vi "Set Number of Slots.vi"(8 "error in":errorcluster, 10 "number of slots":i32, 11 "chassis ref in":T1 format="%.0x") -> (0 "error out":errorcluster, 3 "chassis ref out":T1 format="%.0x")   [LabVIEW 2020, in "Scan Engine Scripting.lvlib"]
doc: "Writes <B>number of slots</B> into the provided chassis reference and edits the existing slots of the chassis to comply with the new limit."
uses:
  Scan Engine Scripting.lvlib
  <vilib>/NI VeriStand/Custom Device API/Custom Device Item Ref.ctl
  Modules.lvlibp/RSI Module/Slot Settings.ctl
  Modules.lvlibp/RSI Module/Module Models.ctl
  Scan Engine Dependencies.llb/Scan Engine GUIDs.vi
  Modules.lvlibp/RSI Module/Class Property Strings.vi
  Scan Engine Dependencies.llb/Property Strings.vi
  <vilib>/NI VeriStand/Custom Device API/Set Item Property (I32).vi
  Scan Engine Dependencies.llb/Scan Engine Custom Device.lvlib
  <vilib>/NI VeriStand/Custom Device API/Custom Device API.lvlib
  Modules.lvlibp/RSI Module/RSI Module.lvclass
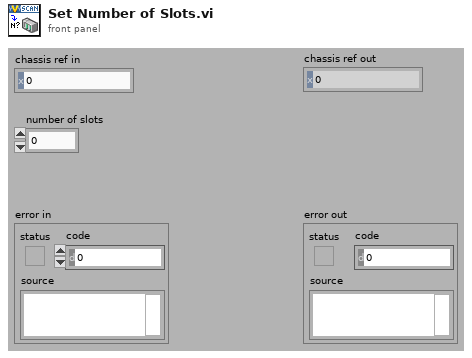
[diagram p1: front panel]
types:
  T1 = typedef "Custom Device API.lvlib/Custom Device Item Ref.ctl" = u64
  T2 = typedef "Modules.lvlibp/RSI Module.lvclass/Module Models.ctl" = enum16{"Empty", "NI 9201", "NI 9203", "NI 9205", "NI 9206", "NI 9207", "NI 9208", "NI 9209", "NI 9210", "NI 9211", "NI 9212", "NI 9213", "NI 9214", "NI 9215", "NI 9216", "NI 9217", "NI 9219", "NI 9220", "NI 9221", "NI 9222", "NI 9223", "NI 9224", "NI 9225", "NI 9226", "NI 9227", "NI 9228", "NI 9229", "NI 9233", "NI 9234", "NI 9235", "NI 9236", "NI 9237", "NI 9239", "NI 9242", "NI 9244", "NI 9253", "NI 9263", "NI 9264", "NI 9265", "NI 9266", "NI 9269", "NI 9344", "NI 9350", "NI 9375", "NI 9401", "NI 9402", "NI 9403", "NI 9411", "NI 9421", "NI 9422", "NI 9423", "NI 9425", "NI 9426", "NI 9435", "NI 9436", "NI 9437", "NI 9472", "NI 9474", "NI 9475", "NI 9476", "NI 9477", "NI 9478", "NI 9481", "NI 9482", "NI 9485"}
  T3 = typedef "Modules.lvlibp/RSI Module.lvclass/Slot Settings.ctl" = cluster{"Slot":u32, "EtherCAT?":bool}
  T4 = typedef "Custom Device API.lvlib/Custom Device Item Info.ctl" = cluster{"Name":string, "Is Channel":bool, "GUID":string, "Is Waveform":bool}
  T5 = typedef "Modules.lvlibp/Custom Device API.lvlib/Custom Device Item Ref.ctl" = u64
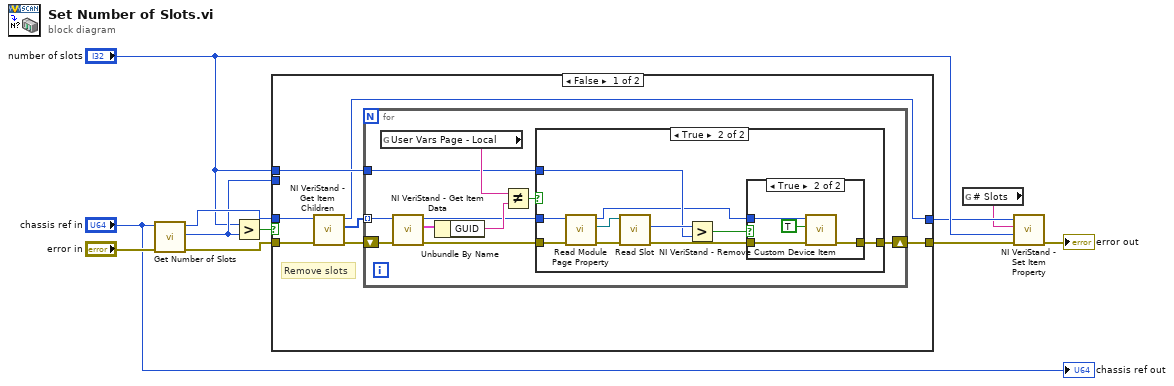
[diagram p0: block diagram]
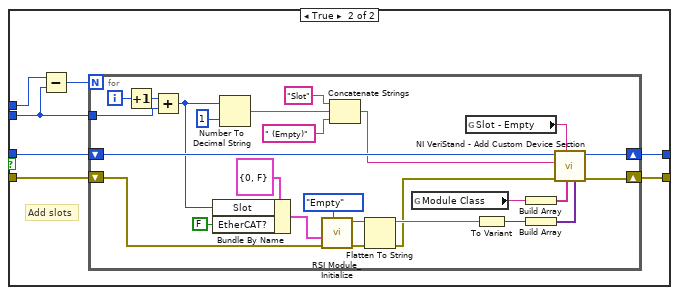
[diagram p4: hidden frame]
diagram:
  n1 = call "Get Number of Slots.vi"("error in"="error in", "chassis ref in"="chassis ref in") -> ("error out"=w11:errorcluster, "number of slots"=w7:i32, "chassis ref out"=w10:T1)  [unwired: 7 in]
  n2 = Greater?(x="number of slots", y=w7) -> (0:w9:bool)
  n3 = case shown="False" w9 {
    tunnel: w10 -> [w18 w47]
    tunnel: w11 -> [w17 w50]
    tunnel: [w14 w46] -> w6
    tunnel: "number of slots" -> [w13 w51]
    tunnel: w7 -> [_ w48]
    tunnel: [w12 w45] -> w3
    frame False {
      # "Remove slots"
      n4 = call <vilib>:"NI VeriStand - Get Item Children.vi"("error in (no error)"=w17, "Item Ref in"=w18) -> ("error out"=w15:errorcluster, "Child Refs"=w16:T1[], "Item Ref out"=w12:T1)  [unwired: 6 in, 1 out]
      n5 = for {
        tunnel: w16 -> [w27] mode=indexing
        shift-right: [w19] -> w14
        shift-left: w15 -> [w28]
        tunnel: w13 -> [w20]
        n6 = global read "Scan Engine GUIDs.vi" "User Vars Page - Local"() -> (w24:string)
        n7 = call <vilib>:"NI VeriStand - Get Item Data.vi"("error in (no error)"=w28, "Item Ref in"=w27) -> ("error out"=w21:errorcluster, "Item Info"=w26:T4, "Item Ref out"=w22:T1)  [unwired: 6 in, 1 out]
        n8 = Unbundle By Name(w26) -> ("GUID"=w25:string)
        n9 = Not Equal?(x=w24, y=w25) -> (x != y?=w23:bool)
        n10 = case shown="True" w23 {
          tunnel: w22 -> [_ w38]
          tunnel: w21 -> [w29 w39]
          tunnel: w20 -> [_ w34]
          tunnel: [w29 w30] -> w19
          frame False {
          }
          frame True {
            n11 = call "Read Module Page Property.vi"("error in (no error)"=w39, "Node Ptr In"=w38) -> ("error out"=w37:errorcluster, "RSI Module"=w36:refnum<class "RSI Module.lvclass">, "Node Ptr Out"=w31:T5)  [unwired: 7 in]
            n12 = call "Read Slot.vi"("error in (no error)"=w37, "RSI Module in"=w36) -> ("error out"=w32:errorcluster, "Slot"=w35:u32)  [unwired: 7 in, 1 out]
            n13 = Greater?(x=w35, y=w34) -> (0:w33:bool)
            n14 = case shown="True" w33 {
              tunnel: w32 -> [w40 w44]
              tunnel: w31 -> [_ w43]
              tunnel: [w40 w41] -> w30
              frame False {
              }
              frame True {
                n15 = call <vilib>:"NI VeriStand - Remove Custom Device Item.vi"("error in (no error)"=w44, "Force Delete (F)"=TRUE, "Item Ref in"=w43) -> ("error out"=w41:errorcluster)  [unwired: 7 in, 1 out]
              }
            }
          }
        }
      }
    }
    frame True {
      # "Add slots"
      n16 = Subtract(x=w51, y=w48) -> (x-y=w49:i32)
      n17 = for {
        N: w49 -> [_]
        shift-right: [w72] -> w46
        shift-left: w50 -> [w65]
        shift-right: [w71] -> w45
        shift-left: w47 -> [w77]
        tunnel: w48 -> [w53]
        i -> [w74]
        n18 = Increment(x=w74) -> (x+1=w54:i32)
        n19 = Add(x=w54, y=w53) -> (x+y=w52:i32)
        n20 = Bundle By Name(cluster=T3 {"Slot"=0, "EtherCAT?"=FALSE} ("Slot Settings"), "Slot"=w52, "EtherCAT?"=FALSE) -> (w68:T3)
        n21 = Number To Decimal String(number=w52, width (-)=i16 1) -> (decimal integer string=w76:string)
        n22 = call "RSI Module_Initialize.vi"("Module Model"=Module_Models."Empty" ("Module"), "error in (no error)"=w65, "Slot Settings"=w68) -> ("error out"=w58:errorcluster, "RSI Module out"=w60:refnum<class "RSI Module.lvclass">)  [unwired: 7 in]
        n23 = Concatenate Strings("Slot" ("string"), w76, " (Empty)" ("Section Name")) -> (w73:string)
        n24 = Flatten To String(anything=w60, error in (no error)=w58) -> (data string=w59:string, error out=w57:errorcluster)  [unwired: 2 in, 1 out]
        n25 = global read "Class Property Strings.vi" "Module Class"() -> (w56:string)
        n26 = global read "Scan Engine GUIDs.vi" "Slot - Empty"() -> (w61:string)
        n27 = To Variant(anything=w59) -> (Variant=w69:variant)
        n28 = Build Array(w56) -> (w64:string[])
        n29 = Build Array(w69) -> (w70:variant[])
        n30 = call <vilib>:"NI VeriStand - Add Custom Device Section.vi"("Property Values"=w70, "Property names"=w64, "GUID (Default Section)"=w61, "error in (no error)"=w57, "Section Name"=w73, "Parent Ref in"=w77) -> ("error out"=w72:errorcluster, "Parent Ref out"=w71:T1)  [unwired: 2 in, 2 out]
      }
    }
  }
  n31 = global read "Property Strings.vi" "# Slots"() -> (w2:string)
  n32 = call-poly <vilib>:"NI VeriStand - Set Item Property.vi"("error in (no error)"=w6, "Value"="number of slots", "Property Name"=w2, "Item Ref in"=w3) -> ("error out"=→"error out":errorcluster)  [unwired: 5 in, 2 out]
  "chassis ref out" <- "chassis ref in"
